vi "FT10_Config Bundle Arrays.vi"(8 "error in (no error)":errorcluster, 10 "String Values Array":string[](array[string]), 11 "Values Found Array":bool[](array[boolean])) -> (0 "error out":errorcluster, 2 "Config String Value Cluster":T5, 3 "Config Keys Found Cluster":T1)   [LabVIEW 2015]
doc: "Bundle boolean and string arrays into clusters"
uses:
  Controls/Control_Config Str Val Cluster.ctl
  Controls/Control_Config Unitherm Str Val.ctl
  Controls/Control_Config Simulation Str Val.ctl
  Controls/Control_Config Fornax Attempts Str Val.ctl
  Controls/Control_Config Keys Found Cluster.ctl
  Controls/Control_Config Unitherm Found Bool.ctl
  Controls/Control_Config Simulation Found Bool.ctl
  Controls/Control_Config Fornax Attempts Found Bool.ctl
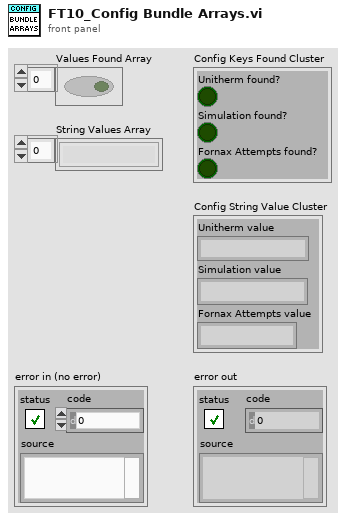
[diagram p1: front panel]
types:
  T1 = typedef "Control_Config Keys Found Cluster.ctl" = cluster{"Unitherm found?":T2, "Simulation found?":T3, "Fornax Attempts found?":T4}
  T2 = typedef "Control_Config Unitherm Found Bool.ctl" = bool
  T3 = typedef "Control_Config Simulation Found Bool.ctl" = bool
  T4 = typedef "Control_Config Fornax Attempts Found Bool.ctl" = bool
  T5 = typedef "Control_Config Str Val Cluster.ctl" = cluster{"Unitherm value":T6, "Simulation value":T7, "Fornax Attempts value":T8}
  T6 = typedef "Control_Config Unitherm Str Val.ctl" = string
  T7 = typedef "Control_Config Simulation Str Val.ctl" = string
  T8 = typedef "Control_Config Fornax Attempts Str Val.ctl" = string
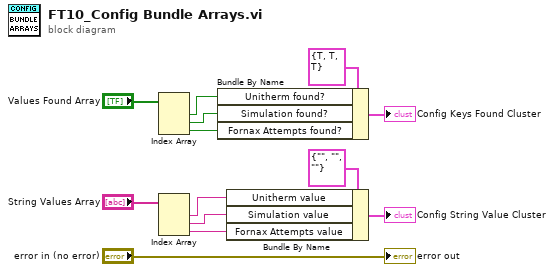
[diagram p0: block diagram]
diagram:
  n1 = Index Array(array="Values Found Array") -> (element #1=w3:bool, element #2=w4:bool, element #3=w5:bool)  [unwired: 3 in]
  n2 = Index Array(array="String Values Array") -> (element #1=w9:string, element #2=w10:string, element #3=w11:string)  [unwired: 3 in]
  n3 = Bundle By Name(cluster=T1 {"Unitherm found?"=TRUE, "Simulation found?"=TRUE, "Fornax Attempts found?"=TRUE}, "Unitherm found?"=w3, "Simulation found?"=w4, "Fornax Attempts found?"=w5) -> (→"Config Keys Found Cluster":T1)
  n4 = Bundle By Name(cluster=T5 {"Unitherm value"="", "Simulation value"="", "Fornax Attempts value"=""}, "Unitherm value"=w9, "Simulation value"=w10, "Fornax Attempts value"=w11) -> (→"Config String Value Cluster":T5)
  "error out" <- "error in (no error)"
